vi "GFGTranslator__WRAPPER.vi"(6 "GFGTranslator Datatype":T2, 7 "GFG Translator Action":T3, 8 "Boolean_Input":bool, 9 "Numeric_Input":dbl, 10 "String_Input":string, 11 "GFG Variable Name":string) -> (0 "I16_2DArray_Output":i16[][](array[numeric]), 1 "Boolean_Output":bool, 2 "Numeric_Output":dbl, 3 "String_Output":string, 4 "Variant_Output":variant, 5 "Status Output":T1)   [LabVIEW 2012]
uses:
  GFGTranslator_Action.ctl
  GFGTranslator_Datatype.ctl
  GFGTranslator_errors.ctl
  <vilib>/Utility/error.llb/whitespace.ctl
panel:
  out "error out":errorcluster
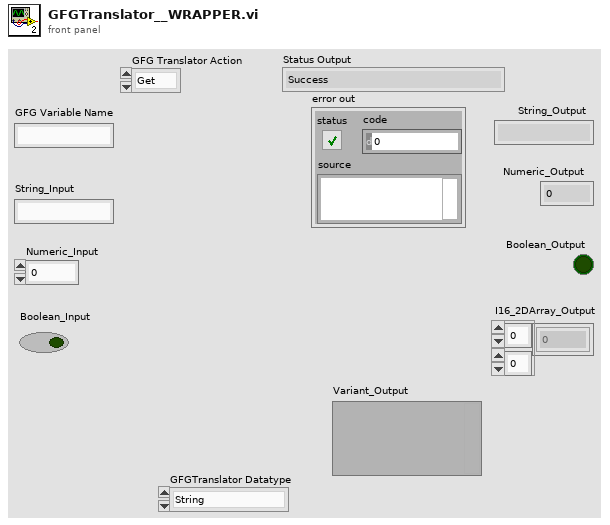
[diagram p1: front panel]
types:
  T1 = typedef "GFGTranslator_errors.ctl" = enum16{"Success", "SciScan Not Running", "No Get Method for Selected Datatype", "No Set Method for Selected Datatype", "Variable Not Found", "Unexpected Datatype", "Data Out of Range"}
  T2 = typedef "GFGTranslator_Datatype.ctl" = enum16{"String", "Path (String)", "Numeric", "Boolean", "Set_BoolRef (use boolean data)", "Get_Variant", "Get_2DArray (I16)", "Get_Image_2DArray (I16)", "Get_Version (String)", "Get_All GFG variables (String)"}
  T3 = typedef "GFGTranslator_Action.ctl" = enum16{"Get", "Set"}
  T4 = typedef "whitespace.ctl" = u16
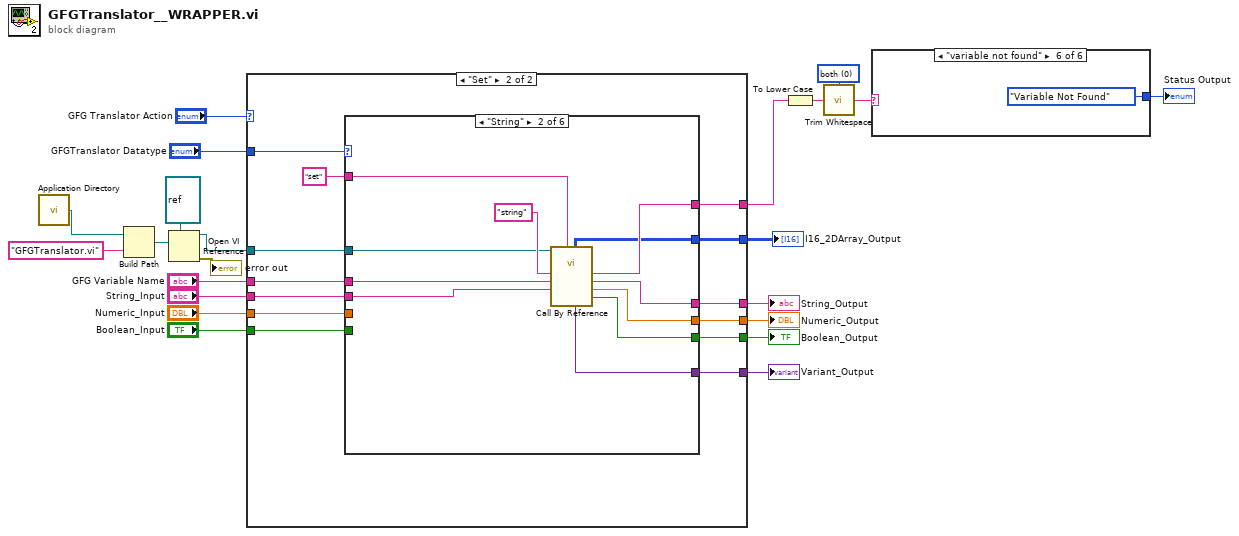
[diagram p0: block diagram]
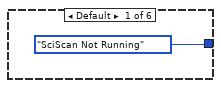
[diagram p2: hidden frame]
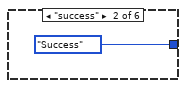
[diagram p3: hidden frame]
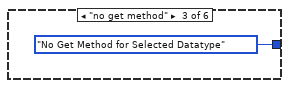
[diagram p4: hidden frame]
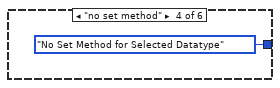
[diagram p5: hidden frame]
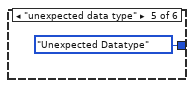
[diagram p6: hidden frame]
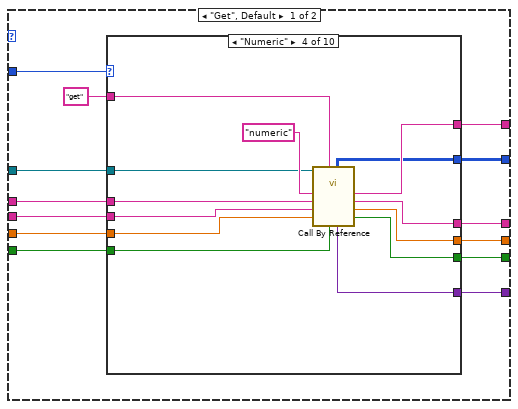
[diagram p7: hidden frame]
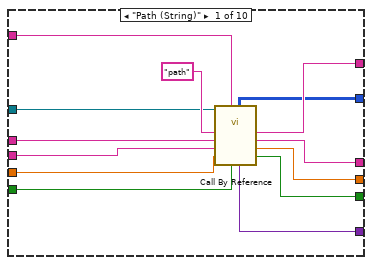
[diagram p8: hidden frame]
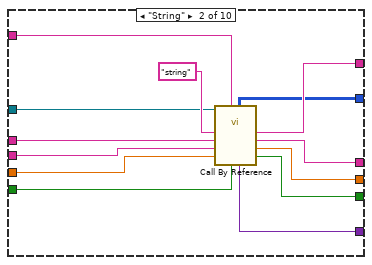
[diagram p9: hidden frame]
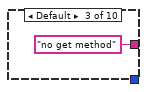
[diagram p10: hidden frame]
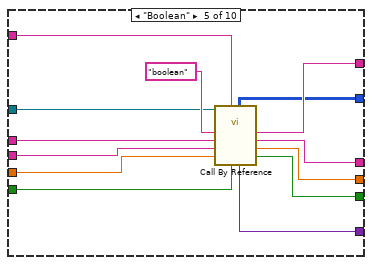
[diagram p11: hidden frame]
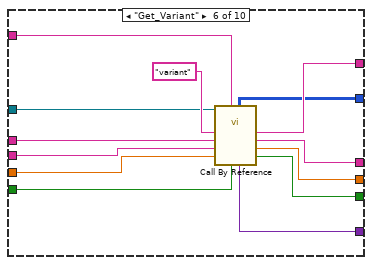
[diagram p12: hidden frame]
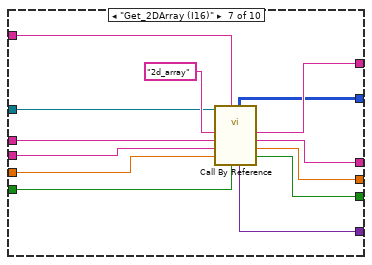
[diagram p13: hidden frame]
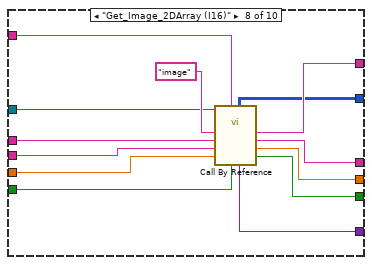
[diagram p14: hidden frame]
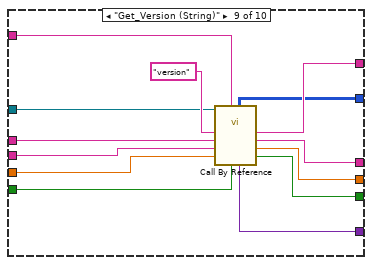
[diagram p15: hidden frame]
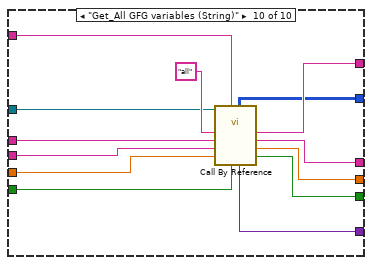
[diagram p16: hidden frame]
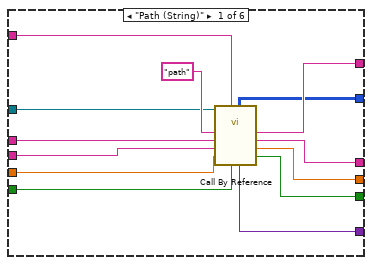
[diagram p17: hidden frame]
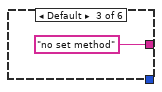
[diagram p18: hidden frame]
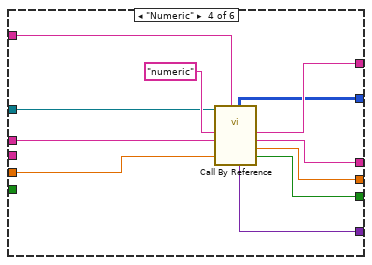
[diagram p19: hidden frame]
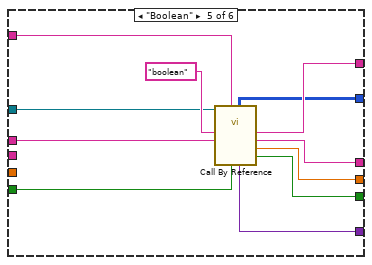
[diagram p20: hidden frame]
diagram:
  w7 = T4 0 items=["both", "start of string", "end of string"] ("location (both)")
  n1 = call <vilib>:"Application Directory.vi"() -> ("Application Directory"=w1:path)
  n2 = Build Path(base path=w1, name or relative path="GFGTranslator.vi") -> (appended path=w17:path)
  n3 = Open VI Reference(type specifier VI Refnum (for type only)=refnum<vi> refnum, vi path=w17) -> (vi reference=w19:refnum<vi>, error out=→"error out":errorcluster)  [unwired: 4 in]
  n4 = case shown="\"Set\"" "GFG Translator Action" {
    tunnel: "GFGTranslator Datatype" -> [w35 w166]
    tunnel: w19 -> [w34 w165]
    tunnel: "GFG Variable Name" -> [w23 w164]
    tunnel: [w32 w162] -> w5
    tunnel: [w31 w161] -> w15
    tunnel: "String_Input" -> [w30 w160]
    tunnel: "Numeric_Input" -> [w29 w159]
    tunnel: "Boolean_Input" -> [w28 w158]
    tunnel: [w27 w157] -> w11
    tunnel: [w26 w156] -> w10
    tunnel: [w25 w155] -> w9
    tunnel: [w24 w154] -> w8
    frame "Get", Default {
      n5 = case shown="\"Numeric\"" w35 {
        tunnel: w34 -> [w36 w49 _ w63 w76 w89 w102 w115 w128 w141]
        tunnel: w23 -> [w47 w60 _ w74 w87 w100 w113 w126 w139 w152]
        tunnel: "get" ("Action") -> [w46 w59 _ w73 w86 w99 w112 w125 w138 w151]
        tunnel: [w45 w58 "no get method" ("status") w72 w85 w98 w111 w124 w137 w150] -> w32
        tunnel: [w44 w57 _ w71 w84 w97 w110 w123 w136 w149] -> w31
        tunnel: w30 -> [w43 w56 _ w70 w83 w96 w109 w122 w135 w148]
        tunnel: w29 -> [w41 w51 _ w69 w82 w95 w108 w121 w134 w147]
        tunnel: w28 -> [w42 w50 _ w68 w81 w94 w107 w120 w133 w146]
        tunnel: [w38 w55 _ w67 w80 w93 w106 w119 w132 w145] -> w27
        tunnel: [w37 w54 _ w66 w79 w92 w105 w118 w131 w144] -> w26
        tunnel: [w39 w52 _ w65 w78 w91 w104 w117 w130 w143] -> w25
        tunnel: [w40 w53 _ w64 w77 w90 w103 w116 w129 w142] -> w24
        frame "Path (String)" {
          n6 = call-by-ref "?"(reference=w36, "boolean_ip"=w42, "Action"=w46, "numeric_ip"=w41, "string_ip"=w43, "GFG_var_name"=w47, "DataType"="path") -> ("boolean_op"=w37:bool, "numeric_op"=w38:dbl, "string_op"=w44:string, "status"=w45:string, "variant_op"=w40:variant, "array_op"=w39:i16[][])  [unwired: 1 in, 2 out]
        }
        frame "String" {
          n7 = call-by-ref "?"(reference=w49, "boolean_ip"=w50, "Action"=w59, "numeric_ip"=w51, "string_ip"=w56, "GFG_var_name"=w60, "DataType"="string") -> ("boolean_op"=w54:bool, "numeric_op"=w55:dbl, "string_op"=w57:string, "status"=w58:string, "variant_op"=w53:variant, "array_op"=w52:i16[][])  [unwired: 1 in, 2 out]
        }
        frame Default {
        }
        frame "Numeric" {
          n8 = call-by-ref "?"(reference=w63, "boolean_ip"=w68, "Action"=w73, "numeric_ip"=w69, "string_ip"=w70, "GFG_var_name"=w74, "DataType"="numeric") -> ("boolean_op"=w66:bool, "numeric_op"=w67:dbl, "string_op"=w71:string, "status"=w72:string, "variant_op"=w64:variant, "array_op"=w65:i16[][])  [unwired: 1 in, 2 out]
        }
        frame "Boolean" {
          n9 = call-by-ref "?"(reference=w76, "boolean_ip"=w81, "Action"=w86, "numeric_ip"=w82, "string_ip"=w83, "GFG_var_name"=w87, "DataType"="boolean") -> ("boolean_op"=w79:bool, "numeric_op"=w80:dbl, "string_op"=w84:string, "status"=w85:string, "variant_op"=w77:variant, "array_op"=w78:i16[][])  [unwired: 1 in, 2 out]
        }
        frame "Get_Variant" {
          n10 = call-by-ref "?"(reference=w89, "boolean_ip"=w94, "Action"=w99, "numeric_ip"=w95, "string_ip"=w96, "GFG_var_name"=w100, "DataType"="variant") -> ("boolean_op"=w92:bool, "numeric_op"=w93:dbl, "string_op"=w97:string, "status"=w98:string, "variant_op"=w90:variant, "array_op"=w91:i16[][])  [unwired: 1 in, 2 out]
        }
        frame "Get_2DArray (I16)" {
          n11 = call-by-ref "?"(reference=w102, "boolean_ip"=w107, "Action"=w112, "numeric_ip"=w108, "string_ip"=w109, "GFG_var_name"=w113, "DataType"="2d_array") -> ("boolean_op"=w105:bool, "numeric_op"=w106:dbl, "string_op"=w110:string, "status"=w111:string, "variant_op"=w103:variant, "array_op"=w104:i16[][])  [unwired: 1 in, 2 out]
        }
        frame "Get_Image_2DArray (I16)" {
          n12 = call-by-ref "?"(reference=w115, "boolean_ip"=w120, "Action"=w125, "numeric_ip"=w121, "string_ip"=w122, "GFG_var_name"=w126, "DataType"="image") -> ("boolean_op"=w118:bool, "numeric_op"=w119:dbl, "string_op"=w123:string, "status"=w124:string, "variant_op"=w116:variant, "array_op"=w117:i16[][])  [unwired: 1 in, 2 out]
        }
        frame "Get_Version (String)" {
          n13 = call-by-ref "?"(reference=w128, "boolean_ip"=w133, "Action"=w138, "numeric_ip"=w134, "string_ip"=w135, "GFG_var_name"=w139, "DataType"="version") -> ("boolean_op"=w131:bool, "numeric_op"=w132:dbl, "string_op"=w136:string, "status"=w137:string, "variant_op"=w129:variant, "array_op"=w130:i16[][])  [unwired: 1 in, 2 out]
        }
        frame "Get_All GFG variables (String)" {
          n14 = call-by-ref "?"(reference=w141, "boolean_ip"=w146, "Action"=w151, "numeric_ip"=w147, "string_ip"=w148, "GFG_var_name"=w152, "DataType"="all") -> ("boolean_op"=w144:bool, "numeric_op"=w145:dbl, "string_op"=w149:string, "status"=w150:string, "variant_op"=w142:variant, "array_op"=w143:i16[][])  [unwired: 1 in, 2 out]
        }
      }
    }
    frame "Set" {
      n15 = case shown="\"String\"" w166 {
        tunnel: w165 -> [w167 w180 _ w192 w203 w214]
        tunnel: w164 -> [w178 w189 _ w201 w212 w223]
        tunnel: "set" ("Action") -> [w177 w188 _ w200 w211 w222]
        tunnel: [w176 w187 "no set method" ("status") w199 w210 w221] -> w162
        tunnel: [w175 w186 _ w198 w209 w220] -> w161
        tunnel: w160 -> [w174 w185 _ _ _ _]
        tunnel: w159 -> [w172 _ _ w197 _ _]
        tunnel: w158 -> [w173 _ _ _ w208 w219]
        tunnel: [w169 w184 _ w196 w207 w218] -> w157
        tunnel: [w168 w183 _ w195 w206 w217] -> w156
        tunnel: [w170 w181 _ w194 w205 w216] -> w155
        tunnel: [w171 w182 _ w193 w204 w215] -> w154
        frame "Path (String)" {
          n16 = call-by-ref "?"(reference=w167, "boolean_ip"=w173, "Action"=w177, "numeric_ip"=w172, "string_ip"=w174, "GFG_var_name"=w178, "DataType"="path") -> ("boolean_op"=w168:bool, "numeric_op"=w169:dbl, "string_op"=w175:string, "status"=w176:string, "variant_op"=w171:variant, "array_op"=w170:i16[][])  [unwired: 1 in, 2 out]
        }
        frame "String" {
          n17 = call-by-ref "?"(reference=w180, "Action"=w188, "string_ip"=w185, "GFG_var_name"=w189, "DataType"="string") -> ("boolean_op"=w183:bool, "numeric_op"=w184:dbl, "string_op"=w186:string, "status"=w187:string, "variant_op"=w182:variant, "array_op"=w181:i16[][])  [unwired: 3 in, 2 out]
        }
        frame Default {
        }
        frame "Numeric" {
          n18 = call-by-ref "?"(reference=w192, "Action"=w200, "numeric_ip"=w197, "GFG_var_name"=w201, "DataType"="numeric") -> ("boolean_op"=w195:bool, "numeric_op"=w196:dbl, "string_op"=w198:string, "status"=w199:string, "variant_op"=w193:variant, "array_op"=w194:i16[][])  [unwired: 3 in, 2 out]
        }
        frame "Boolean" {
          n19 = call-by-ref "?"(reference=w203, "boolean_ip"=w208, "Action"=w211, "GFG_var_name"=w212, "DataType"="boolean") -> ("boolean_op"=w206:bool, "numeric_op"=w207:dbl, "string_op"=w209:string, "status"=w210:string, "variant_op"=w204:variant, "array_op"=w205:i16[][])  [unwired: 3 in, 2 out]
        }
        frame "Set_BoolRef (use boolean data)" {
          n20 = call-by-ref "?"(reference=w214, "boolean_ip"=w219, "Action"=w222, "GFG_var_name"=w223, "DataType"="booleanref") -> ("boolean_op"=w217:bool, "numeric_op"=w218:dbl, "string_op"=w220:string, "status"=w221:string, "variant_op"=w215:variant, "array_op"=w216:i16[][])  [unwired: 3 in, 2 out]
        }
      }
    }
  }
  "String_Output" <- w15
  "Numeric_Output" <- w11
  "Boolean_Output" <- w10
  "Variant_Output" <- w8
  "I16_2DArray_Output" <- w9
  n21 = To Lower Case(string=w5) -> (all lower case string=w4:string)
  n22 = call <vilib>:"Trim Whitespace.vi"("string"=w4, "location (both)"=w7) -> ("trimmed string"=w6:string)
  n23 = case shown="\"variable not found\"" w6 {
    tunnel: [GFGTranslator_errors."SciScan Not Running" ("Ring") GFGTranslator_errors."Success" ("Ring") GFGTranslator_errors."No Get Method for Selected Datatype" ("Ring") GFGTranslator_errors."No Set Method for Selected Datatype" ("Ring") GFGTranslator_errors."Unexpected Datatype" ("Ring") GFGTranslator_errors."Variable Not Found" ("Ring")] -> w3
    frame Default {
    }
    frame "success" {
    }
    frame "no get method" {
    }
    frame "no set method" {
    }
    frame "unexpected data type" {
    }
    frame "variable not found" {
    }
  }
  "Status Output" <- w3
